vi "launch visualizer.vi"(8 "error in (no error)":errorcluster, 11 "Device Ref in":T1 format="%.0x") -> (0 "error out":errorcluster, 3 "reference out":refnum<vi>)   [LabVIEW 2016, in "FPGA Resource Manager.lvlib"]
uses:
  FPGA Resource Manager.lvlib
  <vilib>/NI Veristand/Custom Device API/Custom Device Item Ref.ctl
  <vilib>/NI VeriStand/Custom Device API/Custom Device API.lvlib
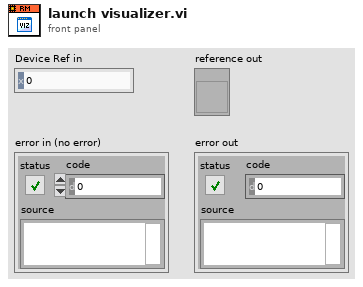
[diagram p1: front panel]
types:
  T1 = typedef "Custom Device API.lvlib/Custom Device Item Ref.ctl" = u64
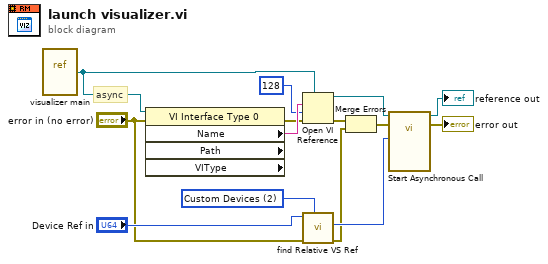
[diagram p0: block diagram]
diagram:
  w6 = u16 2 items=["Targets", "Controller", "Custom Devices", "This CD", "This CD/Group", "This CD/Group/SubGroup"] ("Relative Type")
  # "async"
  n1 = vi-ref "visualizer main.vi"() -> (w14:refnum<vi>)
  n2 = property class="VI Interface Type 0" props=["Name", "Path", "VIType"](reference=w14, error in="error in (no error)") -> (error out=w10:errorcluster, "Name"=w13:string)  [unwired: 3 out]
  n3 = Open VI Reference(type specifier VI Refnum (for type only)=w14, vi path=w13, options=128, error in (no error)=w10) -> (vi reference=w7:refnum<vi>, error out=w4:errorcluster)  [unwired: 2 in]
  n4 = call "find Relative VS Ref.vi"("Relative Type"=w6, "error in (no error)"="error in (no error)", "Item Ref in"="Device Ref in") -> ("error out"=w3:errorcluster, "Relative Item Ref Out"=w5:T1)  [unwired: 4 in, 3 out]
  n5 = Merge Errors(w4, w3) -> (w2:errorcluster)
  n6 = call-by-ref "Start Asynchronous Call"(reference=w7, error in=w2, "Item Ref in"=w5) -> (reference out=→"reference out":refnum<vi>, error out=→"error out":errorcluster)  [unwired: 9 in, 2 out]
